vi "generate filter.vi"(8 "error in (no error)":errorcluster, 9 "filter parameters":T1={"Alpha"=0.5, "Filter Length"=6, "TX Filter"=enum."Root Raised Cos"} {"Alpha" format="%.2f"}, 11 "pulse shaping samples per symbol (16)":i32=16) -> (0 "error out":errorcluster, 1 "matched filter coefficients":dbl[](array[numeric]), 3 "pulse shaping filter coefficients":dbl[](array[numeric]) format="%.2f")   [LabVIEW 2011]
uses:
  FilterCoefficient.ctl
panel:
  out "RX matched filter shape":dbl[](graph)
  out "TX pulse shaping filter shape":dbl[](graph)
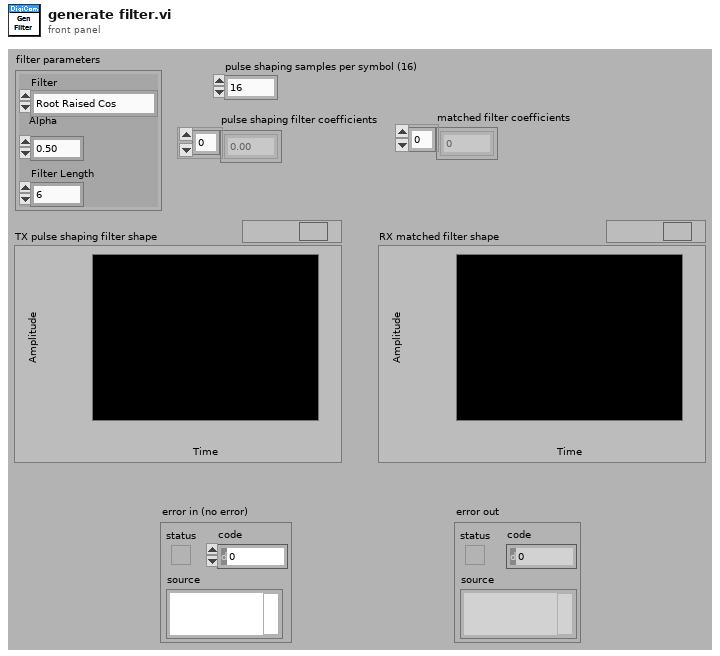
[diagram p1: front panel]
types:
  T1 = typedef "FilterCoefficient.ctl" = cluster{"Alpha":dbl, "Filter Length":i32, "TX Filter":enum16{"Root Raised Cos", "Raised Cos", "Rectangular"}}
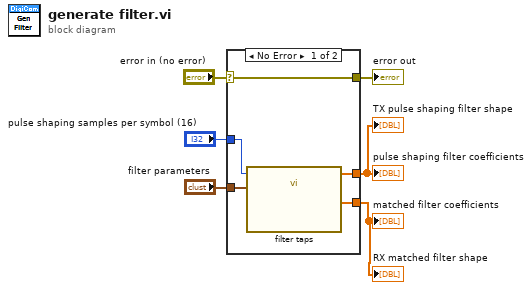
[diagram p0: block diagram]
diagram:
  n1 = case shown="No Error" "error in (no error)" {
    selector: "error in (no error)" -> [w7 w12]
    tunnel: "pulse shaping samples per symbol (16)" -> [w11 _]
    tunnel: [w7 w12] -> w4
    tunnel: [w9 _] -> w3
    tunnel: [w8 _] -> w1
    tunnel: "filter parameters" -> [w10 _]
    frame No Error {
      n2 = call "filter taps.vi"("filter parameters"=w10, "Samples Per Symbol (16)"=w11) -> ("matched filter coefficients"=w8:dbl[], "pulse shaping filter coefficients"=w9:dbl[])  [unwired: 8 in]
    }
    frame Error {
    }
  }
  "error out" <- w4
  "pulse shaping filter coefficients" <- w3
  "TX pulse shaping filter shape" <- w3
  "matched filter coefficients" <- w1
  "RX matched filter shape" <- w1
